vi "Post-Build Action.vi"(5 "Files Generated by Build":path[](array[path]), 6 "Top Level/Always Included VIs":path[](array[path]), 7 "Destination Path":path, 8 "error in (no error)":errorcluster, 9 "Target Name":string, 10 "Build Specification Name":string, 11 "Project Path":path) -> (0 "error out":errorcluster)   [LabVIEW 2015, in "BuildVIs.lvlib"]
uses:
  BuildVIs.lvlib
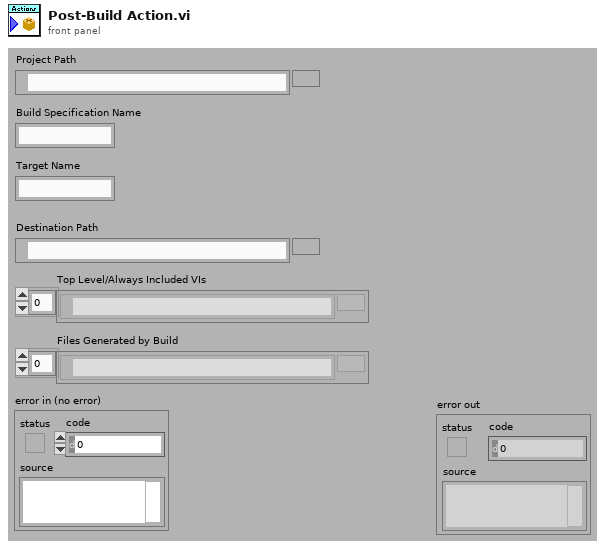
[diagram p1: front panel]
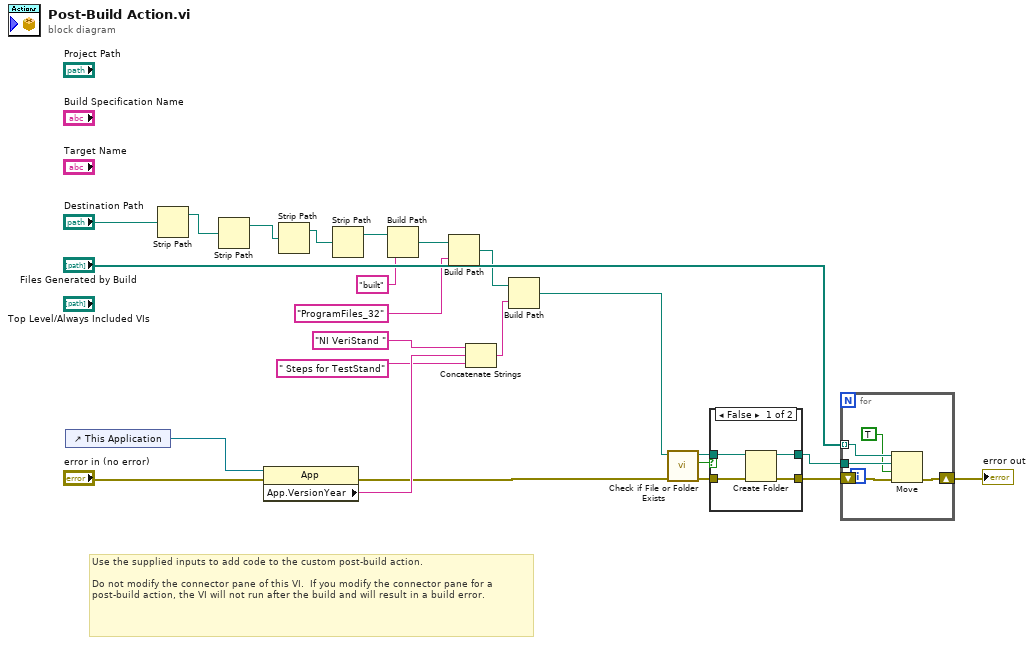
[diagram p0: block diagram]
diagram:
  # "Use the supplied inputs to add code to the custom post-build action.\n\nDo not modify the connector pane of this VI.  If you modify the connector pane for a post-build action, the VI will not run after the build and will result in a build error."
  n1 = control-ref of="This Application"() -> (w7:refnum<vi>)
  n2 = Strip Path(path="Destination Path") -> (stripped path=w16:path)  [unwired: 1 out]
  n3 = Strip Path(path=w16) -> (stripped path=w15:path)  [unwired: 1 out]
  n4 = property class="App"(reference=w7, error in="error in (no error)") -> (error out=w1:errorcluster, "App.VersionYear"=w5:string)  [unwired: 1 out]
  n5 = Strip Path(path=w15) -> (stripped path=w14:path)  [unwired: 1 out]
  n6 = Strip Path(path=w14) -> (stripped path=w13:path)  [unwired: 1 out]
  n7 = Build Path(base path=w13, name or relative path="built") -> (appended path=w11:path)
  n8 = Build Path(base path=w11, name or relative path="ProgramFiles_32") -> (appended path=w9:path)
  n9 = Concatenate Strings("NI VeriStand " ("name or relative path"), w5, " Steps for TestStand" ("string")) -> (w3:string)
  n10 = Build Path(base path=w9, name or relative path=w3) -> (appended path=w8:path)
  n11 = call <vilib>:"Check if File or Folder Exists.vi"("error in (no error)"=w1, "path"=w8) -> ("error out"=w24:errorcluster, "file or folder exists?"=w23:bool, "dup path"=w22:path)  [unwired: 7 in]
  n12 = case shown="False" w23 {
    tunnel: w24 -> [w28 w29]
    tunnel: w22 -> [w26 w30]
    tunnel: [w27 w29] -> w21
    tunnel: [w25 w30] -> w19
    frame False {
      n13 = Create Folder(path (use dialog)=w26, error in=w28) -> (created path=w25:path, error out=w27:errorcluster)  [unwired: 1 in, 1 out]
    }
    frame True {
    }
  }
  n14 = for {
    tunnel: w19 -> [w33]
    shift-right: [w34] -> w20
    shift-left: w21 -> [w35]
    tunnel: "Files Generated by Build" -> [w32] mode=indexing
    n15 = Move(source path=w32, error in=w35, 9:TRUE ("overwrite (F)"), 10:w33) -> (error out=w34:errorcluster)  [unwired: 1 in, 2 out]
  }
  "error out" <- w20
